vi "Check Multicast IP.vi"(11 "net address":u32 format="%.0x") -> (2 "Broadcast":bool, 3 "Multicast":bool)   [LabVIEW 2021, in "Networking_CIF_U.lvlib"]
uses:
  Networking_CIF_U.lvlib
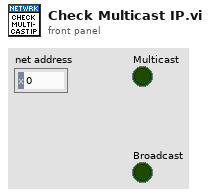
[diagram p1: front panel]
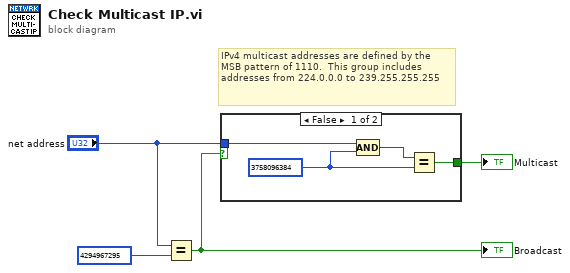
[diagram p0: block diagram]
diagram:
  # "IPv4 multicast addresses are defined by the MSB pattern of 1110.  This group includes addresses from 224.0.0.0 to 239.255.255.255"
  n1 = Equal?(x="net address", y=u32 4294967295 ("value")) -> (x = y?=w1:bool)
  "Broadcast" <- w1
  n2 = case shown="False" w1 {
    tunnel: [w7 _] -> w4
    tunnel: "net address" -> [w5 _]
    frame False {
      w6 = u32 3758096384 ("value")
      n3 = Compound Arithmetic op=AND(w5, w6) -> (w8:u32)
      n4 = Equal?(x=w8, y=w6) -> (x = y?=w7:bool)
    }
    frame True {
    }
  }
  "Multicast" <- w4
